vi "CANOpen_NMT_Setup NG.vi"(7 "Node ID":u8, 8 "error in":errorcluster, 10 "Period":u16, 11 "interface object in":refnum<k20>) -> (0 "error out":errorcluster, 3 "interface object out":refnum<k20>)   [LabVIEW 2021, in "CANOpen Addon Engine.lvlib"]
uses:
  <vilib>/CANopenLib/CANOPEN.llb/CANopen SDO Create.vi
  <vilib>/CANopenLib/CANOPEN.llb/CANopen SDO Write [U16].vi
  <vilib>/CANopenLib/CANOPEN.llb/CANopen SDO Write [U8].vi
  <vilib>/CANopenLib/CANOPEN.llb/CANopen SDO Close.vi
  CANOpen Addon Engine.lvlib
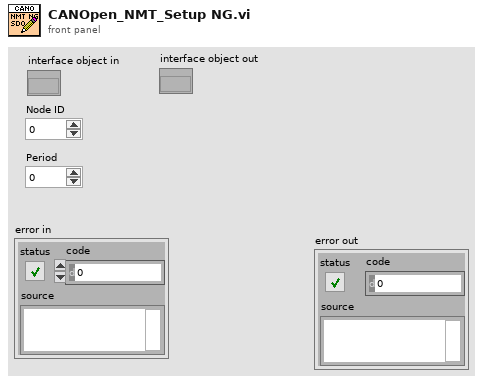
[diagram p1: front panel]
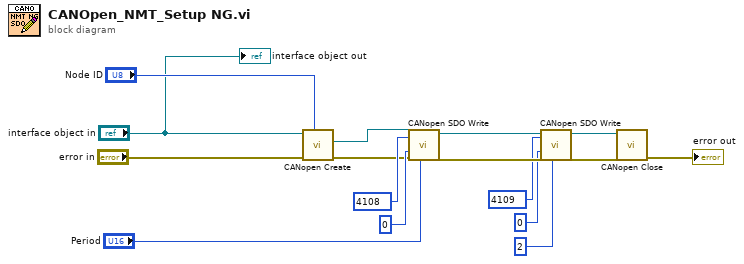
[diagram p0: block diagram]
diagram:
  n1 = call-poly <vilib>:"CANopen Create.vi"("node-ID"="Node ID", "error in (no error)"="error in", "interface object in"="interface object in") -> ("error out"=w3:errorcluster, "SDO object out"=w2:refnum<k20>)  [unwired: 6 in, 1 out]
  n2 = call-poly <vilib>:"CANopen SDO Write.vi"("U16 data"="Period", "error in (no error)"=w3, "object sub-index (0)"=u8 0, "object index"=u16 4108, "SDO object in"=w2) -> ("error out"=w10:errorcluster, "SDO object out"=w8:refnum<k20>)  [unwired: 4 in, 1 out]
  n3 = call-poly <vilib>:"CANopen SDO Write.vi"("U8 data"=u8 2, "error in (no error)"=w10, "object sub-index (0)"=u8 0, "object index"=u16 4109, "SDO object in"=w8) -> ("error out"=w11:errorcluster, "SDO object out"=w9:refnum<k20>)  [unwired: 4 in, 1 out]
  n4 = call-poly <vilib>:"CANopen Close.vi"("error in (no error)"=w11, "SDO object in"=w9) -> ("error out"=→"error out":errorcluster)  [unwired: 9 in]
  "interface object out" <- "interface object in"
